vi "Senkenregler_PID.vi"(0 "Regelventil 36":dbl, 1 "Time Target (s)":dbl=60.0, 2 "Auto Reset":bool=TRUE, 3 "Schaltprozent":dbl=1.0, 5 "Solltemp.":dbl=43.0 format="%.2f", 7 "Regelventil 35":dbl, 9 "?":T1={"proportional gain (Kc)"=2.8, "integral time (Ti, min)"=1.0, "derivative time (Td, min)"=0.0} {"derivative time (Td, min)" format="%.3f"; "integral time (Ti, min)" format="%.3f"; "proportional gain (Kc)" format="%.3f"}, 11 "Regler Senke":bool, 12 "reinitialize?":bool, 13 "RV 36  Regeld.":dbl=0.5, 14 "TI_35":dbl) -> (4 "upper limit 2":dbl, 6 "upper limit":dbl, 8 "Regeldifferenz 2":dbl, 10 "Reglerausgabe":dbl)   [LabVIEW 2015]
uses:
  <vilib>/addons/control/pid/pid.llb/PID (DBL).vi
  <vilib>/addons/control/pid/NI_PID_pid.lvlib
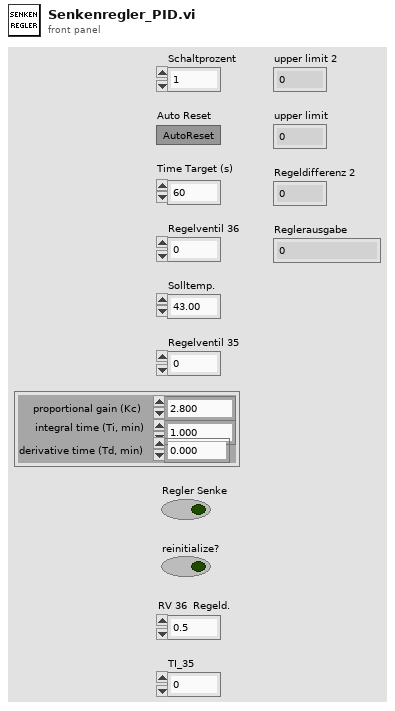
[diagram p1: front panel]
types:
  T1 = cluster{"proportional gain (Kc)":dbl, "integral time (Ti, min)":dbl, "derivative time (Td, min)":dbl}
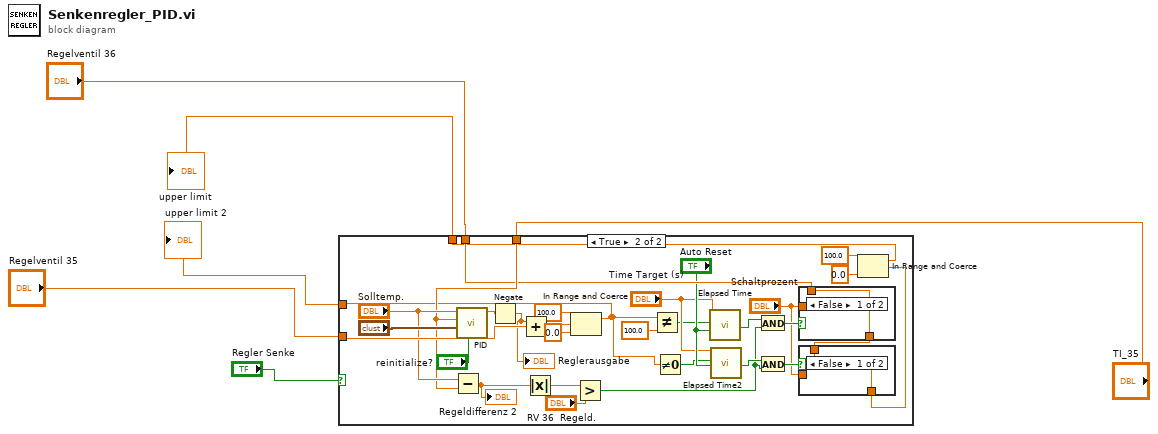
[diagram p0: block diagram]
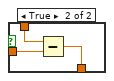
[diagram p3: hidden frame]
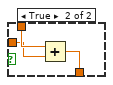
[diagram p4: hidden frame]
diagram:
  n1 = case shown="True" "Regler Senke" {
    tunnel: [w8 w12] -> w3
    tunnel: "Regelventil 35" -> [w8 w37]
    tunnel: "TI_35" -> [_ w35]
    tunnel: "Regelventil 36" -> [w7 w24]
    tunnel: [w7 w17] -> w5
    frame False {
    }
    frame True {
      n2 = Subtract(x="Solltemp.", y=w35) -> (x-y=w32:dbl)
      "Regeldifferenz 2" <- w32
      n3 = call-poly <vilib>:"PID.vi"("reinitialize? (F)"="reinitialize?", "PID gains"="?", "process variable"=w35, "setpoint"="Solltemp.") -> ("output"=w10:dbl)  [unwired: 6 in, 1 out]
      n4 = Negate(x=w10) -> (-x=w9:dbl)
      "Reglerausgabe" <- w9
      n5 = Add(x=w9, y=w37) -> (x+y=w11:dbl)
      n6 = Absolute Value(x=w32) -> (abs(x)=w31:dbl)
      n7 = In Range and Coerce(upper limit=100.0, x=w11, lower limit=0.0) -> (coerced(x)=w12:dbl)  [unwired: 1 out]
      n8 = Greater?(x=w31, y="RV 36  Regeld.") -> (0:w27:bool)
      n9 = Not Equal?(x=w12, y=100.0) -> (x != y?=w14:bool)
      n10 = Not Equal To 0?(x=w12) -> (x != 0?=w13:bool)
      n11 = call "Elapsed Time"("Time Target (s)"="Time Target (s)", "Reset"=w14, "Auto Reset"="Auto Reset") -> ("Time has Elapsed"=w29:bool)  [unwired: 9 in, 7 out]
      n12 = call "Elapsed Time2"("Time Target (s)"="Time Target (s)", "Reset"=w13, "Auto Reset"="Auto Reset") -> ("Time has Elapsed"=w28:bool)  [unwired: 9 in, 7 out]
      n13 = And(x=w29, y=w27) -> (x .and. y?=w26:bool)
      n14 = And(x=w28, y=w27) -> (x .and. y?=w25:bool)
      n15 = case shown="False" w26 {
        tunnel: w24 -> [w44 w47]
        tunnel: [w44 w46] -> w23
        tunnel: "Schaltprozent" -> [_ w45]
        frame False {
        }
        frame True {
          n16 = Add(x=w47, y=w45) -> (x+y=w46:dbl)
        }
      }
      n17 = case shown="False" w25 {
        tunnel: [w40 w42] -> w18
        tunnel: w23 -> [w40 w43]
        tunnel: "Schaltprozent" -> [_ w41]
        frame False {
        }
        frame True {
          n18 = Subtract(x=w43, y=w41) -> (x-y=w42:dbl)
        }
      }
      n19 = In Range and Coerce(upper limit=100.0, x=w18, lower limit=0.0) -> (coerced(x)=w17:dbl)  [unwired: 1 out]
    }
  }
  "upper limit" <- w5
  "upper limit 2" <- w3
